vi "SwerveChooseBestAngle.vi"(5 "Goal Override":bool, 7 "Goal Override Angle (deg) [-180,+180]":dbl format="%#_13g", 8 "Hysteresis (deg)":dbl=10.0 format="%#_13g", 10 "Goal Angle (deg) [-180,+180]":dbl format="%#_13g", 11 "Current Angle (deg) [-180,+180]":dbl format="%#_13g") -> (0 "Flip Drive Motor Direction":bool, 2 "Flipped Angular Distance (deg)":dbl format="%_4g", 3 "Flipped Goal Angle (deg) [-180, +180]":dbl)   [LabVIEW 2020]
doc: "Based on the Current Angle and the Goal Angle, this VI calulates the signed angular distance. Taking into account the option to invert the direction of the swerve drive motor and always picking the shortest travel distance. The hysteresis prevents undesirable vacillation between angle choices."
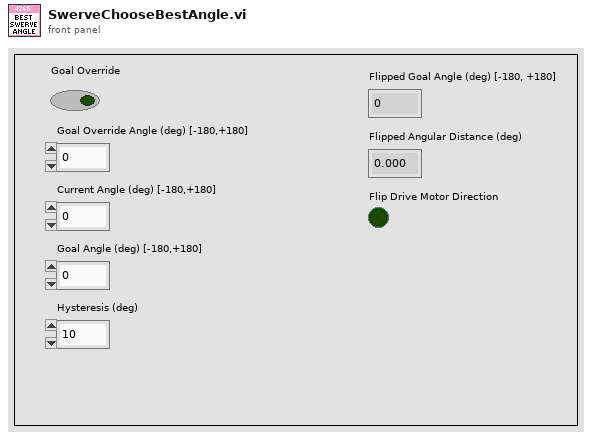
[diagram p1: front panel]
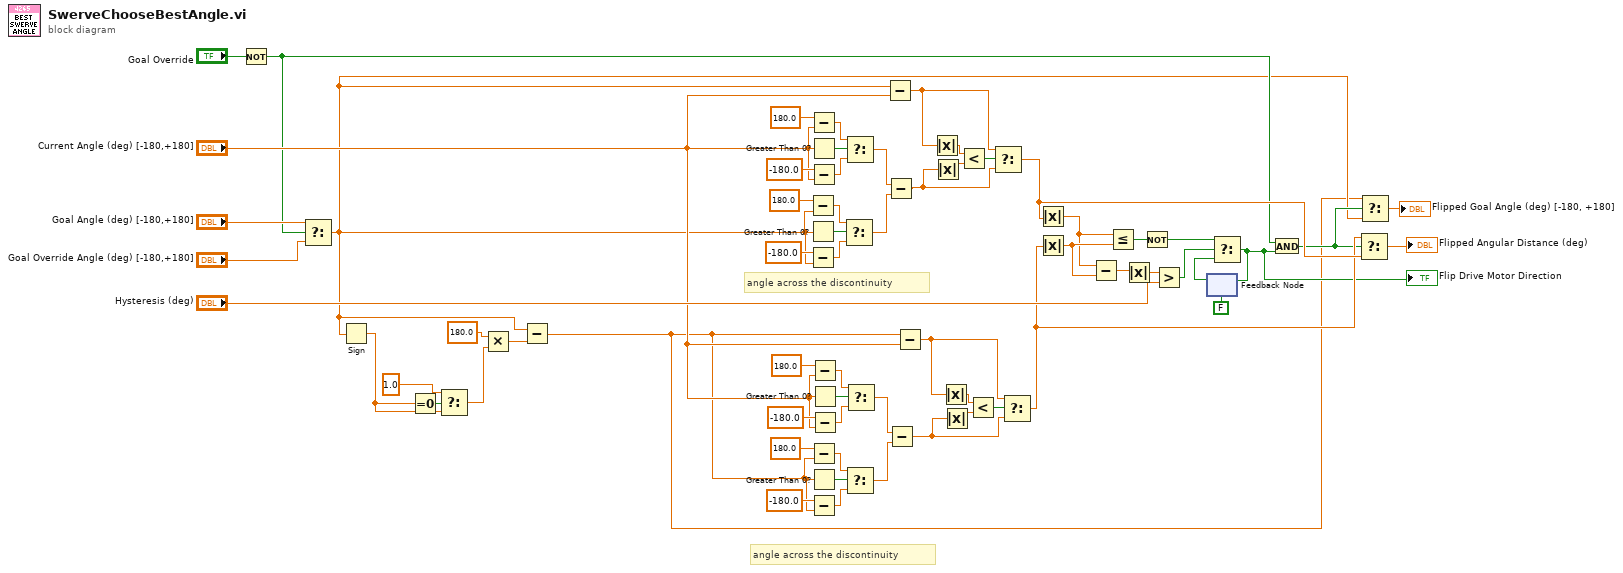
[diagram p0: block diagram]
diagram:
  # "angle across the discontinuity"
  # "angle across the discontinuity"
  n1 = Not(x="Goal Override") -> (.not. x?=w6:bool)
  n2 = Select(t="Goal Angle (deg) [-180,+180]", s=w6, f="Goal Override Angle (deg) [-180,+180]") -> (s? t:f=w3:dbl)
  n3 = Sign(1:w3) -> (0:w15:dbl)
  n4 = Equal To 0?(x=w15) -> (x = 0?=w16:bool)
  n5 = Select(t=1.0, s=w16, f=w15) -> (s? t:f=w12:dbl)
  n6 = Multiply(x=180.0 ("y"), y=w12) -> (x*y=w63:dbl)
  n7 = Subtract(x=w3, y=w63) -> (x-y=w2:dbl)
  n8 = Subtract(x=180.0, y=w3) -> (x-y=w25:dbl)
  n9 = Greater Than 0?(x=w3) -> (x > 0?=w27:bool)
  n10 = Subtract(x=-180.0, y=w3) -> (x-y=w23:dbl)
  n11 = Subtract(x=180.0, y="Current Angle (deg) [-180,+180]") -> (x-y=w30:dbl)
  n12 = Greater Than 0?(x="Current Angle (deg) [-180,+180]") -> (x > 0?=w32:bool)
  n13 = Subtract(x=-180.0, y="Current Angle (deg) [-180,+180]") -> (x-y=w28:dbl)
  n14 = Subtract(x=180.0, y=w2) -> (x-y=w45:dbl)
  n15 = Greater Than 0?(x=w2) -> (x > 0?=w47:bool)
  n16 = Subtract(x=-180.0, y=w2) -> (x-y=w43:dbl)
  n17 = Subtract(x=180.0, y="Current Angle (deg) [-180,+180]") -> (x-y=w51:dbl)
  n18 = Greater Than 0?(x="Current Angle (deg) [-180,+180]") -> (x > 0?=w53:bool)
  n19 = Subtract(x=-180.0, y="Current Angle (deg) [-180,+180]") -> (x-y=w49:dbl)
  n20 = Select(t=w25, s=w27, f=w23) -> (s? t:f=w21:dbl)
  n21 = Select(t=w30, s=w32, f=w28) -> (s? t:f=w22:dbl)
  n22 = Select(t=w45, s=w47, f=w43) -> (s? t:f=w41:dbl)
  n23 = Select(t=w51, s=w53, f=w49) -> (s? t:f=w42:dbl)
  n24 = Subtract(x=w3, y="Current Angle (deg) [-180,+180]") -> (x-y=w33:dbl)
  n25 = Subtract(x=w22, y=w21) -> (x-y=w19:dbl)
  n26 = Subtract(x=w42, y=w41) -> (x-y=w40:dbl)
  n27 = Subtract(x=w2, y="Current Angle (deg) [-180,+180]") -> (x-y=w37:dbl)
  n28 = Absolute Value(x=w33) -> (abs(x)=w34:dbl)
  n29 = Absolute Value(x=w19) -> (abs(x)=w35:dbl)
  n30 = Absolute Value(x=w37) -> (abs(x)=w38:dbl)
  n31 = Absolute Value(x=w40) -> (abs(x)=w39:dbl)
  n32 = Less?(x=w34, y=w35) -> (x < y?=w36:bool)
  n33 = Less?(x=w38, y=w39) -> (x < y?=w48:bool)
  n34 = Select(t=w33, s=w36, f=w19) -> (s? t:f=w11:dbl)
  n35 = Select(t=w37, s=w48, f=w40) -> (s? t:f=w10:dbl)
  n36 = Absolute Value(x=w11) -> (abs(x)=w54:dbl)
  n37 = Absolute Value(x=w10) -> (abs(x)=w55:dbl)
  n38 = Subtract(x=w54, y=w55) -> (x-y=w59:dbl)
  n39 = Less Or Equal?(x=w54, y=w55) -> (x <= y?=w18:bool)
  n40 = Absolute Value(x=w59) -> (abs(x)=w58:dbl)
  n41 = Not(x=w18) -> (.not. x?=w17:bool)
  n42 = Greater?(x=w58, y="Hysteresis (deg)") -> (0:w56:bool)
  n43 = feedback #1(FALSE) -> (w61:bool)
  n44 = Select(t=w17, s=w56, f=w61) -> (s? t:f=w9:bool)
  "Flip Drive Motor Direction" <- w9
  n45 = feedback-in #1(w9) -> ()
  n46 = And(x=w6, y=w9) -> (x .and. y?=w4:bool)
  n47 = Select(t=w10, s=w4, f=w11) -> (s? t:f=→"Flipped Angular Distance (deg)":dbl)
  n48 = Select(t=w2, s=w4, f=w3) -> (s? t:f=→"Flipped Goal Angle (deg) [-180, +180]":dbl)
